vi "Documentation.vi"() -> (0 "Author":string, 1 "History":string, 2 "Version":string, 3 "Description":string)   [LabVIEW 2021, in "Template_Plugin.lvlib"]
uses:
  Template_Plugin.lvlib
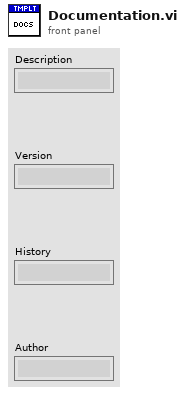
[diagram p1: front panel]
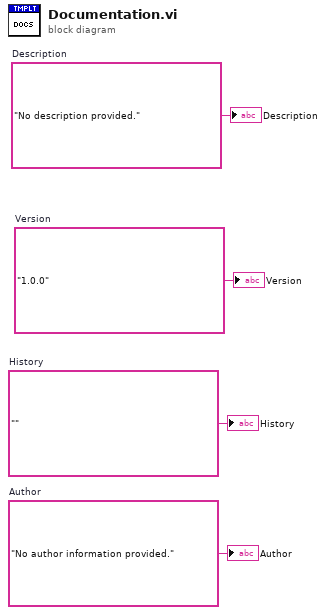
[diagram p0: block diagram]
diagram:
  w1 = "No author information provided."  # Author
  w2 = ""  # History
  w3 = "1.0.0"  # Version
  w4 = "No description provided."  # Description
  "Description" <- w4
  "Version" <- w3
  "History" <- w2
  "Author" <- w1
